vi "Phasor Check Gated Decay Calculation Flags.vi"(9 "Analytical Computation?":bool, 10 "Gate/IRF Type":T1, 11 "Gate Width: W":ext) -> (1 "Square Gate?":bool, 3 "Analytical?":bool)   [LabVIEW 2021, in "Phasor.lvlib"]
uses:
  Phasor.lvlib
  Phasor Gate Type.ctl
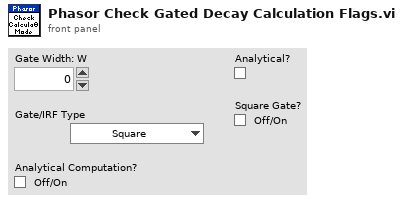
[diagram p1: front panel]
types:
  T1 = typedef "Phasor.lvlib/Phasor Gate Type.ctl" = enum16{"Square", "Finite Edge Square", "Finite Edge, Tilted Top Square", "Triangle", "Sawtooth", "User-defined"}
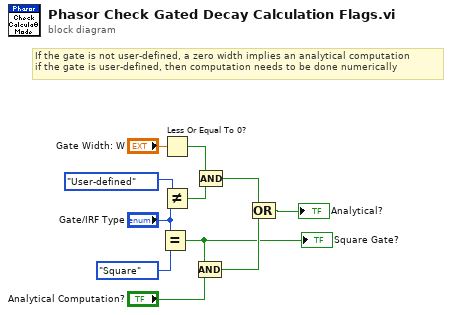
[diagram p0: block diagram]
diagram:
  # "If the gate is not user-defined, a zero width implies an analytical computation\nif the gate is user-defined, then computation needs to be done numerically"
  n1 = Equal?(x="Gate/IRF Type", y=Phasor_Gate_Type."Square" ("Gate Type")) -> (x = y?=w8:bool)
  "Square Gate?" <- w8
  n2 = Less Or Equal To 0?(x="Gate Width: W") -> (x <= 0?=w3:bool)
  n3 = Not Equal?(x=Phasor_Gate_Type."User-defined", y="Gate/IRF Type") -> (x != y?=w2:bool)
  n4 = Compound Arithmetic op=AND(w8, "Analytical Computation?") -> (w11:bool)
  n5 = Compound Arithmetic op=AND(w3, w2) -> (w1:bool)
  n6 = Compound Arithmetic op=OR(w1, w11) -> (→"Analytical?":bool)
